vi "Disabled state-Speed graph behaviour ctrl.vi"(8 "error in (no error)":errorcluster, 10 "Disabled":T1(ring)) -> (0 "error out":errorcluster)   [LabVIEW 2013]
uses:
  Patch-Vol video generator/Globals/gl_8-bit montage window ctrl refs.vi
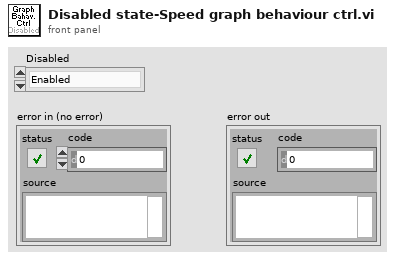
[diagram p1: front panel]
types:
  T1 = enum8{"Enabled", "Disabled", "Disabled and Grayed Out"}
  T2 = typedef "8-bit video export window ctrl refs.ctl" = cluster{"Add speed data":refnum<vi>, "Add camera videos":refnum<vi>, "Stop button":refnum<vi>, "Camera Video Adjustments":refnum<vi>, "Microscope Image Adjustments":refnum<vi>, "Execute":refnum<vi>, "Codec":refnum<vi>, "Channel":refnum<vi>, "Speed graph behaviour":refnum<vi>, "Include speed graph":refnum<vi>}
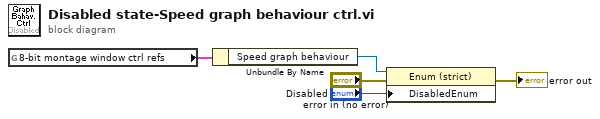
[diagram p0: block diagram]
diagram:
  n1 = global read "gl_8-bit montage window ctrl refs.vi" "8-bit montage window ctrl refs"() -> (w1:T2)
  n2 = Unbundle By Name(w1) -> ("Speed graph behaviour"=w2:refnum<vi>)
  n3 = property on="Property Node" class="Enum (strict)"(reference=w2, error in="error in (no error)", "DisabledEnum"="Disabled") -> (error out=→"error out":errorcluster)  [unwired: 1 out]
